vi "GetStringGlobalVariable.vi"(8 "error in (no error)":errorcluster, 10 "varNumber":i32, 11 "controller in":refnum<k24>) -> (0 "error out":errorcluster, 2 "string value out":string, 3 "controller out":refnum<k24>)   [LabVIEW 2020, in "Aerotech.lvlib"]
uses:
  Aerotech.lvlib
  C:/Users/HEP/Documents/GitHub/UCSB-Gantry-HEP/Drivers/Aerotech A3200/Bin/Aerotech.A3200.LabVIEW.dll
  UCSB-Gantry-HEP/Drivers/Aerotech A3200/Bin/Aerotech.A3200.LabVIEW.dll
  C:/Program Files (x86)/Aerotech/A3200/LabVIEW/2010/Bin/Aerotech.A3200.dll
  Program Files (x86)/Aerotech/A3200/LabVIEW/2010/Bin/Aerotech.A3200.dll
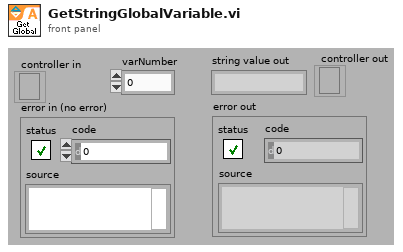
[diagram p1: front panel]
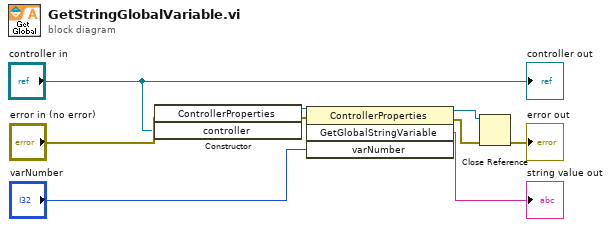
[diagram p0: block diagram]
diagram:
  n1 = constructor class="ControllerProperties"(error in="error in (no error)", "controller"="controller in") -> (reference out=w9:refnum<k24>, error out=w7:errorcluster)  [unwired: 2 in, 2 out]
  n2 = invoke class="ControllerProperties" method="GetGlobalStringVariable"(reference=w9, error in=w7, "varNumber"="varNumber") -> (reference out=w3:refnum<k24>, error out=w1:errorcluster, "GetGlobalStringVariable"=→"string value out":string)  [unwired: 1 in, 1 out]
  n3 = Close Reference(reference=w3, error in (no error)=w1) -> (error out=→"error out":errorcluster)
  "controller out" <- "controller in"
